vi "Fpga-AXI-Stream.vi"() -> ()   [LabVIEW 2017]
uses:
  <vilib>/Platform/TimedLoop/XDataNode/timing_clust.ctl
  <vilib>/Platform/TimedLoop/XDataNode/nitl_modes.ctl
  <vilib>/Platform/TimedLoop/XDataNode/wakeup.ctl
  <vilib>/rvi/Emulation/niFpgaSctlEmulationGetInTimedLoop.vi
  <vilib>/rvi/Emulation/niFpgaEmulationReportErrorSimple.vi
  <vilib>/rvi/Emulation/niFpgaGetClockAttributes.vi
  <vilib>/rvi/Emulation/niFpgaCriticalErrorInLSC.vi
  <vilib>/rvi/eio/common/nirviEmuTemplateMethod_errors.vi
  <vilib>/rvi/interface/RandomDataEmulation/niFpgaRandomDataHandleErrors.vi
  <vilib>/Platform/TimedLoop/XDataNode/XDataNode.xnode
  <vilib>/eio/EIONode/EIONode.xnode
  <vilib>/rvi/DataTransferAndStorage/Container/XNode/niFpgaContainer.xnode
  <vilib>/rvi/interface/RandomDataEmulation/nirviRandomDataFpgaReadWriteTemplate.vi
  <vilib>/Platform/TimedLoop/XDataNode/XDNodeRunTimeDep.lvlib
panel:
  in  "AXI_STR_RXD_tkeep":fxp<+,4,4>
  out "TXD_tuser_count":u32
  out "TXD_tkeep_count":u32
  out "AXI_STR_TXD_tkeep":fxp<+,4,4>
  out "AXI_STR_TXD_tuser":fxp<+,4,4>
  in  "AXI_STR_RXD_tuser":fxp<+,4,4>
  in  "ResetN\n(Active High)":bool
  out "tdata_LastNonZero":u32
  out "tlast_Count":u16
  out "tvalid_Count":u16
  out "AXI_STR_RXD_tready_Count":u16
  out "tlast":bool
  out "tdata":u32
  out "tvalid":bool
  out "AXI_STR_RXD_tready":bool
  out "GPIO #1 out":u32 format="%.0x"
  in  "GPIO #1 in":u32
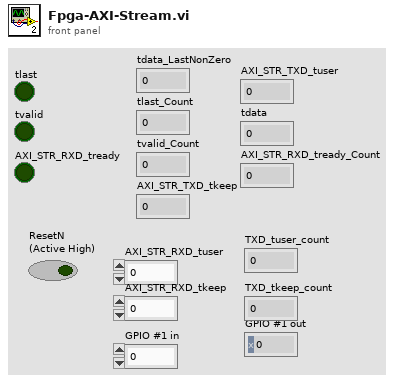
[diagram p1: front panel]
types:
  T1 = typedef "XDNodeRunTimeDep.lvlib/timing_clust.ctl" = cluster{"Expected End [f-1]":u64, "Actual End [f-1]":u64, "Finished Late? [f-1]":bool, "Expected End [i-1]":u64, "Actual End [i-1]":u64, "Finished Late? [i-1]":bool, "Expected Start [i]":u64, "Actual Start [i]":u64, "Expected Start [f]":u64, "Actual Start [f]":u64, "Source Name":string, "Structure Name":string, "Period":i64, "Deadline":i64, "Offset":i64, "Start":i64, "Priority":i32, "Timeout":i32, "Mode":T2, "Wakeup Reason":T3, "Error":errorcluster, "Source Type":string, "Secondary Source Type":string, "Global End Time":u64, "Global Start Time":u64, "Frame Duration":u64, "Iteration Duration":u64, "Assigned CPU":i32, "I/O Scan Engine Mode":u32}
  T2 = typedef "XDNodeRunTimeDep.lvlib/nitl_modes.ctl" = enum32{"No Change", "Process missed periods, maintain original phase", "Discard missed periods, maintain original phase", "Process missed periods, ignore original phase", "Discard missed periods, ignore original phase"}
  T3 = typedef "XDNodeRunTimeDep.lvlib/wakeup.ctl" = enum32{"Normal", "Aborted", "Asynchronous wakeup", "Timing source error", "Timed loop error", "Timeout"}
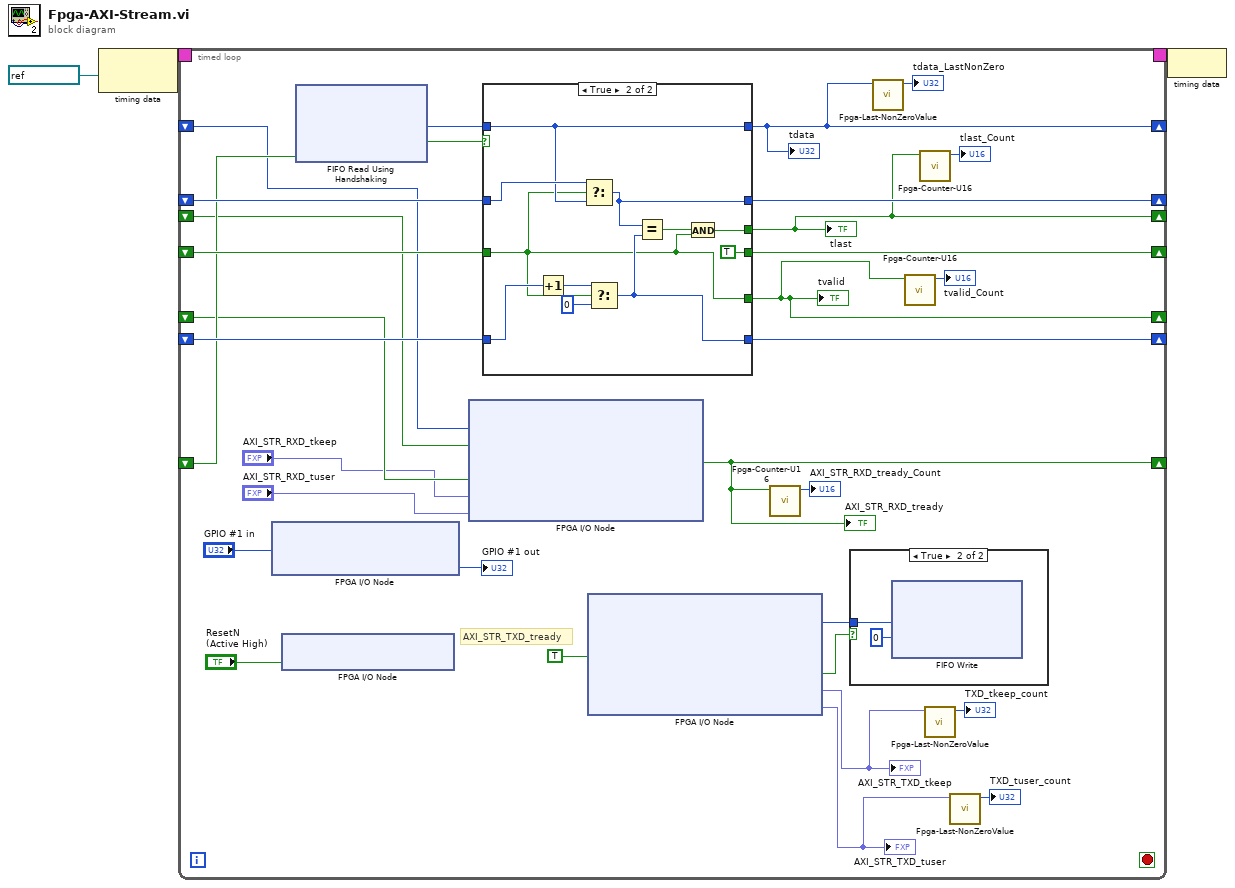
[diagram p0: block diagram]
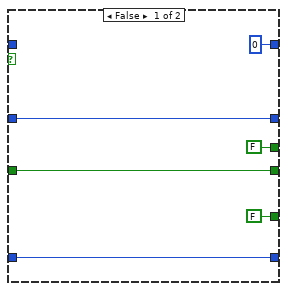
[diagram p3: hidden frame]
diagram:
  n1 = node-c288(refnum<k21> "100MHz" ("Source Name")) -> (w3:T1)
  n2 = timed-loop {
    timing: w3 -> [_]
    timing-out: [_] -> w2
    shift-right: [w33] -> _
    shift-left: _ -> [w34]
    shift-right: [w30] -> _
    shift-left: _ -> [w32]
    shift-right: [w28] -> _
    shift-left: _ -> [w29]
    shift-right: [w25] -> _
    shift-left: _ -> [w10]
    shift-right: [w13] -> _
    shift-left: _ -> [w27]
    shift-right: [w21] -> _
    shift-left: _ -> [w12]
    shift-right: [w23] -> _
    shift-left: _ -> [w11]
    stop <- _ stop-if-true
    # "AXI_STR_TXD_tready"
    n3 = xnode "FPGA I/O Node"("d_microblaze_i\\GPIO1_tri_i"="GPIO #1 in") -> ("d_microblaze_i\\GPIO2_tri_o"=→"GPIO #1 out":u32)  [unwired: 2 in, 2 out]
    n4 = xnode "FPGA I/O Node"("d_microblaze_i\\sys_reset"="ResetN\n(Active High)") -> ()  [unwired: 1 in, 1 out]
    n5 = xnode ("FIFO Read Using Handshaking")("Ready for Output"=w27) -> ("Element"=w31:u32, "Output Valid"=w35:bool)  [unwired: 1 in, 1 out]
    n6 = xnode "FPGA I/O Node"("d_microblaze_i\\AXI_STR_RXD_tdata"=w12, "d_microblaze_i\\AXI_STR_RXD_tlast"=w11, "d_microblaze_i\\AXI_STR_RXD_tvalid"=w10, "d_microblaze_i\\AXI_STR_RXD_tkeep"="AXI_STR_RXD_tkeep", "d_microblaze_i\\AXI_STR_RXD_tuser"="AXI_STR_RXD_tuser") -> ("d_microblaze_i\\AXI_STR_RXD_tready"=w13:bool)  [unwired: 6 in, 6 out]
    "AXI_STR_RXD_tready" <- w13
    n7 = case shown="True" w35 {
      tunnel: w34 -> [w42 w44]
      tunnel: [w42 TRUE ("Size\nRead?")] -> w33
      tunnel: w32 -> [w43 w54]
      tunnel: w31 -> [_ w49]
      tunnel: [w43 w48] -> w30
      tunnel: w29 -> [w41 w53]
      tunnel: [w41 w47] -> w28
      tunnel: [FALSE ("Size\nRead?") w44] -> w25
      tunnel: [u32 0 ("Element") w49] -> w21
      tunnel: [FALSE w45] -> w23
      frame False {
      }
      frame True {
        n8 = Increment(x=w53) -> (x+1=w51:u32)
        n9 = Select(t=w54, s=w44, f=w49) -> (s? t:f=w48:u32)
        n10 = Select(t=w51, s=w44, f=u32 0) -> (s? t:f=w47:u32)
        n11 = Equal?(x=w48, y=w47) -> (x = y?=w46:bool)
        n12 = And(x=w46, y=w44) -> (x .and. y?=w45:bool)
      }
    }
    "tvalid" <- w25
    "tdata" <- w21
    "tlast" <- w23
    n13 = xnode "FPGA I/O Node"("d_microblaze_i\\AXI_STR_TXD_tready"=TRUE ("AXI_STR_TXD_tready")) -> ("d_microblaze_i\\AXI_STR_TXD_tdata"=w16:u32, "d_microblaze_i\\AXI_STR_TXD_tvalid"=w15:bool, "d_microblaze_i\\AXI_STR_TXD_tkeep"=w8:fxp<+,4,4>, "d_microblaze_i\\AXI_STR_TXD_tuser"=w7:fxp<+,4,4>)  [unwired: 6 in, 7 out]
    "AXI_STR_TXD_tuser" <- w7
    "AXI_STR_TXD_tkeep" <- w8
    n14 = call "Fpga-Counter-U16.vi"("d_mcs_i\\IO_BUS_read_strobe"=w13) -> ("Numeric"=→"AXI_STR_RXD_tready_Count":u16)  [unwired: 10 in]
    n15 = case shown="True" w15 {
      tunnel: w16 -> [_ w37]
      frame False {
      }
      frame True {
        n16 = xnode ("FIFO Write")("Element"=w37, "Timeout"=0) -> ()  [unwired: 1 in, 2 out]
      }
    }
    n17 = call "Fpga-Last-NonZeroValue.vi"("d_mcs_i\\IO_BUS_write_data in"=w21) -> ("d_mcs_i\\IO_BUS_write_data out"=→"tdata_LastNonZero":u32)  [unwired: 10 in]
    n18 = call "Fpga-Counter-U16.vi"("d_mcs_i\\IO_BUS_read_strobe"=w25) -> ("Numeric"=→"tvalid_Count":u16)  [unwired: 10 in]
    n19 = call "Fpga-Counter-U16.vi"("d_mcs_i\\IO_BUS_read_strobe"=w23) -> ("Numeric"=→"tlast_Count":u16)  [unwired: 10 in]
    n20 = call "Fpga-Last-NonZeroValue.vi"("d_mcs_i\\IO_BUS_write_data in"=w8) -> ("d_mcs_i\\IO_BUS_write_data out"=→"TXD_tkeep_count":u32)  [unwired: 10 in]
    n21 = call "Fpga-Last-NonZeroValue.vi"("d_mcs_i\\IO_BUS_write_data in"=w7) -> ("d_mcs_i\\IO_BUS_write_data out"=→"TXD_tuser_count":u32)  [unwired: 10 in]
  }
  n22 = node-c288(w2) -> ()
